vi "LVGraphAdd.vi"(7 "Label":string, 8 "error in (no error)":errorcluster, 9 "DataArray":dbl[](array[numeric]), 10 "TimeArray":timestamp[](array[timestamp]), 11 "LVGraph in":refnum<class "LVGraph.lvclass">) -> (0 "error out":errorcluster, 3 "LVGraph out":refnum<class "LVGraph.lvclass">)   [LabVIEW 2017, in "LVGraph.lvclass"]
uses:
  LVGraph.lvclass
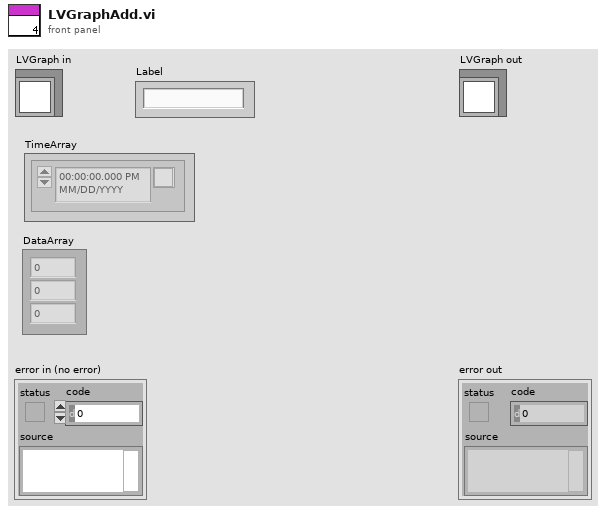
[diagram p1: front panel]
types:
  T1 = cluster{"DataArray":dbl[], "TimeArray":timestamp[]}[][]
  T2 = cluster{"DataArray":dbl[], "TimeArray":timestamp[]}[]
  T3 = cluster{"TimeArray":timestamp[], "DataArray":dbl[]}
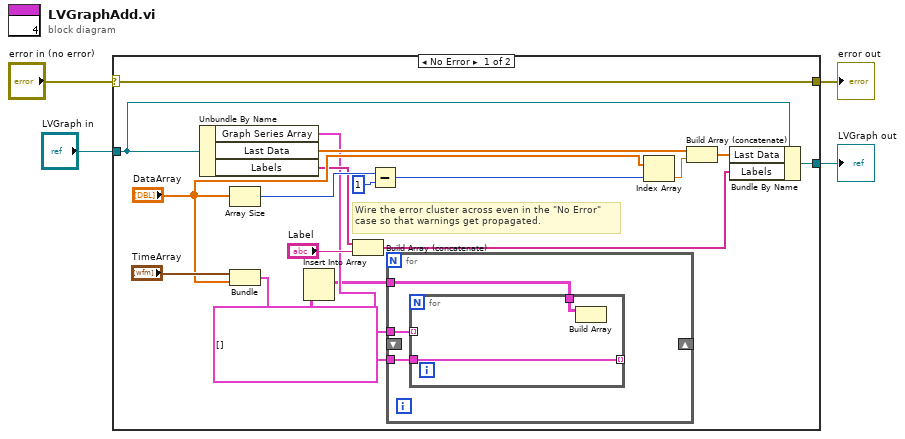
[diagram p0: block diagram]
diagram:
  n1 = case shown="No Error" "error in (no error)" {
    selector: "error in (no error)" -> [w21 w28]
    tunnel: [w21 w28] -> w3
    tunnel: [w12 w27] -> w1
    tunnel: "LVGraph in" -> [w19 w27]
    frame No Error {
      # "Wire the error cluster across even in the \"No Error\"\ncase so that warnings get propagated."
      n2 = Unbundle By Name(w19) -> ("Graph Series Array"=w7:T2, "Last Data"=w18:dbl[], "Labels"=w9:string[])
      n3 = Array Size(array="DataArray") -> (size(s)=w16:i32)
      n4 = Bundle("TimeArray"="TimeArray", "DataArray"="DataArray") -> (w6:T3)  [unwired: 1 in]
      n5 = Insert Into Array() -> ()  [unwired: 3 in, 1 out]
      n6 = Build Array (concatenate)(w9, "Label") -> (w8:string[])
      n7 = Subtract(x=w16, y=1) -> (x-y=w14:i32)
      n8 = for {
        tunnel: w7 -> [w24]
        tunnel: w6 -> [w23]
        shift-right: _ -> [_]
        shift-left: _ -> [_]
        tunnel: T1 [] -> [w22]
        n9 = for {
          tunnel: w24 -> [_] mode=indexing
          tunnel: w23 -> [w26]
          tunnel: [w26] -> _ mode=indexing
          tunnel: w22 -> [w25]
          n10 = Build Array(w25) -> ()  [unwired: 1 in, 1 out]
        }
      }
      n11 = Index Array(array="DataArray", index=w14) -> (element=w13:dbl)
      n12 = Build Array (concatenate)(w18, w13) -> (w11:dbl[])
      n13 = Bundle By Name(cluster=w19, "Last Data"=w11, "Labels"=w8) -> (w12:refnum<class "LVGraph.lvclass">)
    }
    frame Error {
    }
  }
  "error out" <- w3
  "LVGraph out" <- w1
